vi "KillAllModals.vi"() -> ()   [LabVIEW 2018]
doc: "Use this VI standalone to kill all modal windows of a running VI. This is useful during development if in ill-behaving modal VI needs to be shut down via the block diagram.\n\nIn some projects, some VIs may have user controls such as the abort button or close button hidden, so this VI provides a systematic way for the developer to close them without having to exit LabVIEW. \n\nAlso see SetDialogBoxesToModal.vi\n\nCopyright © 2011 Epimedia, Inc. All Rights Reserved.\n\nThe Epimedia Application Library is Copyright © 2009-2011 Epimedia, Inc. \nAll Rights Reserved. Used under license."
panel:
  out "ErrorOut":errorcluster
  in  "ErrorIn":errorcluster
  # "Copyright © 2011 Epimedia, Inc. All Rights Reserved.\n\nThe Epimedia Application Library is Copyright © 2009-2011 Epimedia, Inc. \nAll Rights Reserved. Used under license."
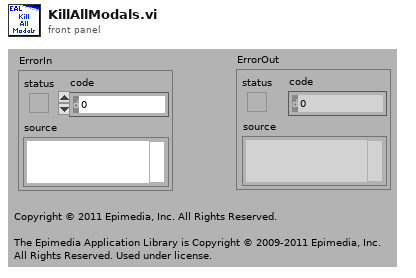
[diagram p1: front panel]
types:
  T1 = enum32{"Invalid", "Default", "Floating", "Floating/Auto-Hide", "Modal"}
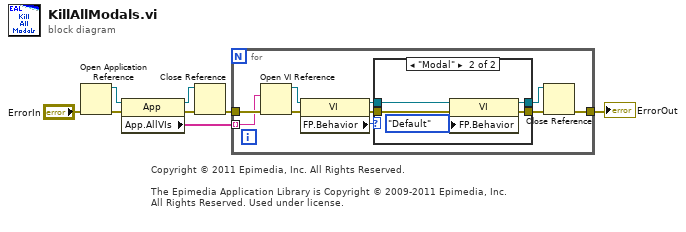
[diagram p0: block diagram]
diagram:
  # "Copyright © 2011 Epimedia, Inc. All Rights Reserved.\n\nThe Epimedia Application Library is Copyright © 2009-2011 Epimedia, Inc. \nAll Rights Reserved. Used under license."
  n1 = Open Application Reference(8:"ErrorIn") -> (0:w8:errorcluster, 3:w7:refnum<vi>)  [unwired: 3 in]
  n2 = property class="App"(reference=w7, error in=w8) -> (reference out=w6:refnum<vi>, error out=w5:errorcluster, "App.AllVIs"=w3:string[])
  n3 = Close Reference(reference=w6, error in (no error)=w5) -> (error out=w4:errorcluster)
  n4 = for {
    tunnel: w3 -> [w17] mode=indexing
    tunnel: w4 -> [w18]
    tunnel: [w9] -> w2
    n5 = Open VI Reference(vi path=w17, error in (no error)=w18) -> (vi reference=w15:refnum<vi>, error out=w16:errorcluster)  [unwired: 4 in]
    n6 = property class="VI"(reference=w15, error in=w16) -> (reference out=w13:refnum<vi>, error out=w12:errorcluster, "FP.Behavior"=w14:T1)
    n7 = case shown="\"Modal\"" w14 {
      tunnel: w13 -> [w20 w25]
      tunnel: w12 -> [w19 w24]
      tunnel: [w19 w22] -> w11
      tunnel: [w20 w21] -> w10
      frame "Default", Default {
      }
      frame "Modal" {
        n8 = property class="VI"(reference=w25, error in=w24, "FP.Behavior"=T1."Default" ("Front Panel Window:Behavior")) -> (reference out=w21:refnum<vi>, error out=w22:errorcluster)
      }
    }
    n9 = Close Reference(reference=w10, error in (no error)=w11) -> (error out=w9:errorcluster)
  }
  "ErrorOut" <- w2
